vi "Measurement setup.vi"() -> ()   [LabVIEW 2016]
uses:
  Modulation_Signals.ctl
  Modulation_types.ctl
  <vilib>/Utility/config.llb/Write Key (String).vi
  <vilib>/Utility/config.llb/Write Key (Double).vi
  <vilib>/Utility/config.llb/Write Key (Path).vi
  <vilib>/Utility/config.llb/Write Key (Boolean).vi
  <vilib>/Utility/config.llb/Write Key (I32).vi
  <vilib>/Utility/file.llb/Write Delimited Spreadsheet (string).vi
  <vilib>/Utility/file.llb/Write Delimited Spreadsheet (DBL).vi
  <vilib>/Utility/config.llb/NI_LVConfig.lvlib
panel:
  in  "Input channels":cluster{string, "physical channels":tag}[](array[cluster])
  in  "Output channels":cluster{string, "physical channels":tag}[](array[cluster])=[{"ao0", "physical channels"="Dev1/ao0"}, {"ao1", "physical channels"="Dev1/ao1"}]
  in  "Signal param 2":dbl format="%#_6p"
  in  "Mearurement range":dbl=5.0 format="%0.2f"
  in  "High cutoff":dbl=20000.0 format="%#_13p"
  in  "Low cutoff":dbl=20.0 format="%#_13p"
  in  "Filter":bool=TRUE
  out "Export path":path
  in  "Export data":bool
  out "Sampling number":i32
  out "Running":bool
  in  "Resampled iterations":dbl=1.0
  in  "File path":path
  in  "Start":bool
  in  "Modulation type":T1=enum."Simple"
  in  "Modulation signal":T2=enum."Sine"
  out "Output":waveform(dbl)[](graph)
  in  "Modulation depth":dbl=0.8 min=0.0 max=1.000001 step=0.1 format="%0.2f"
  in  "Samples":dbl=200.0 format="%#_12g"
  in  "Signal frequency":dbl=1000.0 format="%#_6p"
  in  "Output Fs":dbl=192000.0 format="%#_6p"
  out "Samples per cycle":dbl=10.0
  in  "Carrier frequency":dbl=40000.0 min=0.0 step=1000.0 format="%#_6p"
  out "data":waveform(dbl)[](graph) caption="Input"
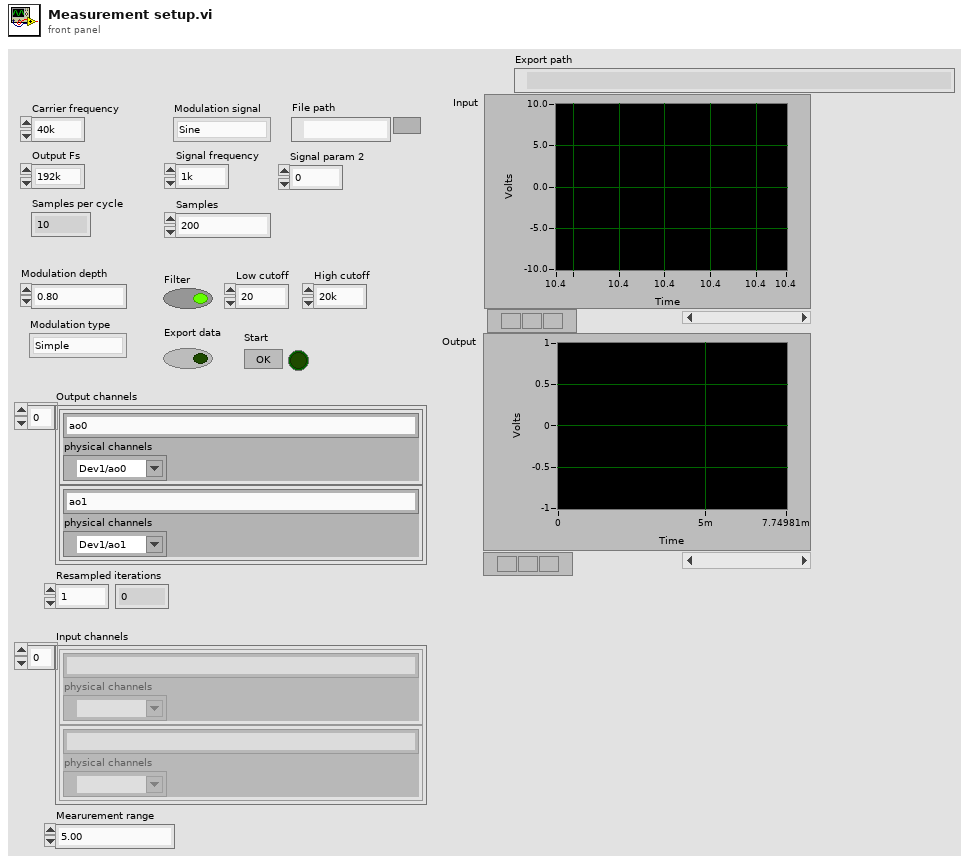
[diagram p1: front panel]
types:
  T1 = typedef "Modulation_types.ctl" = enum16{"None", "Add", "Simple", "Offset", "Square root", "Exponential"}
  T2 = typedef "Modulation_Signals.ctl" = enum16{"None", "Sine", "Chirp", "White Noise", "File"}
  T3 = typedef "NI_LVConfig.lvlib/Config Data RefNum.ctl" = refnum<k1>
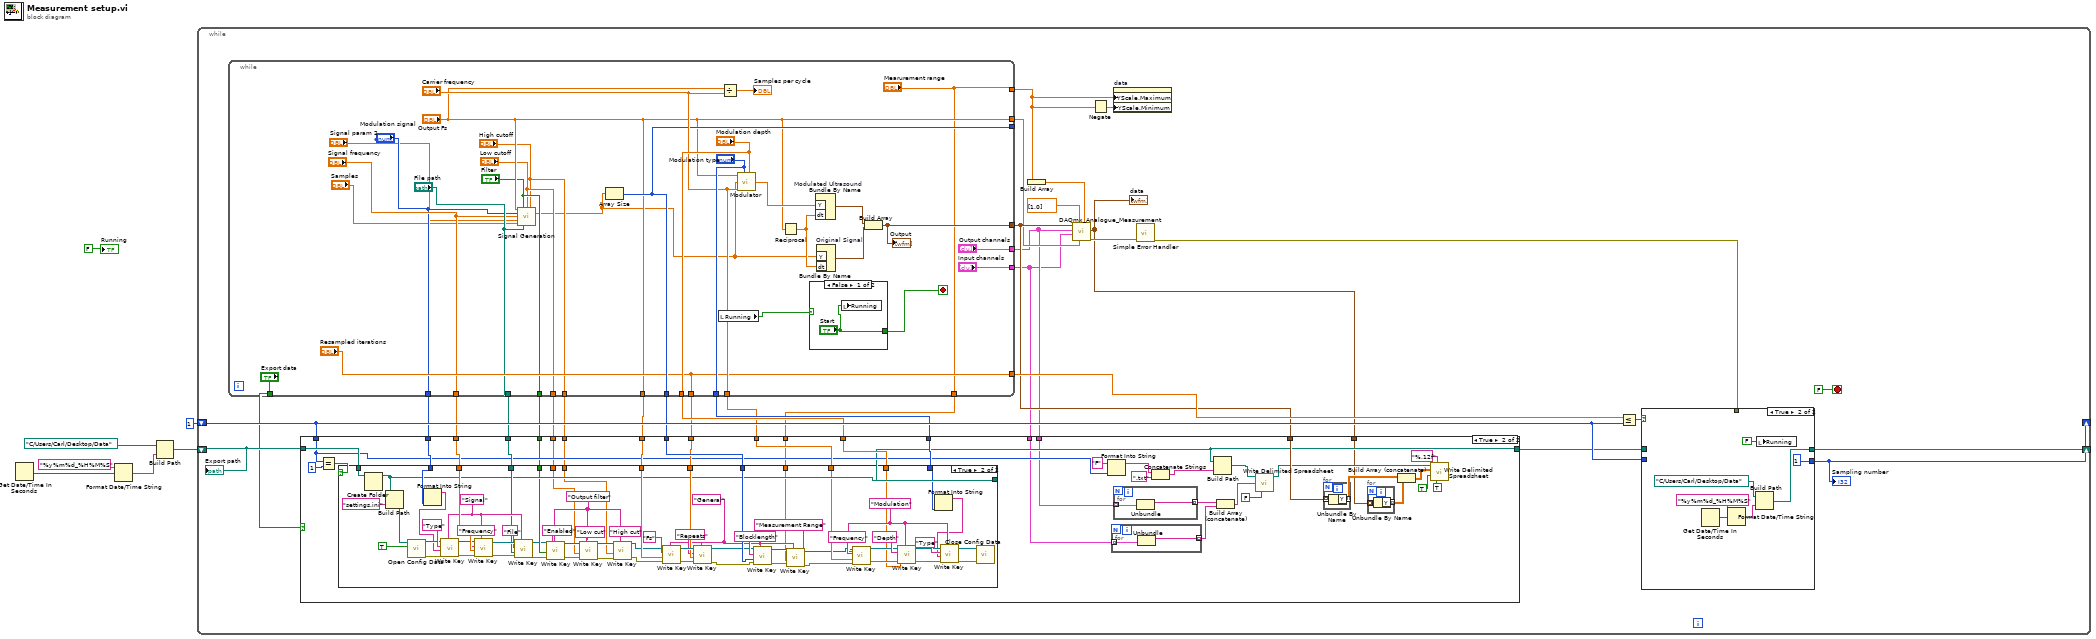
[diagram p0: block diagram]
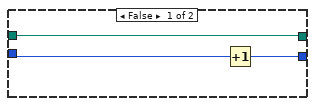
[diagram p4: hidden frame]
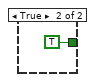
[diagram p5: hidden frame]
diagram:
  n1 = Get Date/Time In Seconds() -> (seconds since 1Jan1904=w6:timestamp)
  n2 = Format Date/Time String(time format string (%c)="%y%m%d_%H%M%S", seconds (now)=w6) -> (date/time string=w5:string)  [unwired: 1 in]
  n3 = Build Path(base path=path "C:/Users/Carl/Desktop/Data", name or relative path=w5) -> (appended path=w2:path)
  n4 = while {
    shift-right: [w39] -> _
    shift-left: 1 ("Sampling number") -> [w38]
    shift-right: [w36] -> _
    shift-left: w2 -> [w35]
    stop <- FALSE stop-if-true
    n5 = while {
      tunnel: [w179] -> _
      tunnel: ["Output Fs"] -> w15
      tunnel: [w187] -> w18
      tunnel: ["Resampled iterations"] -> w19
      tunnel: ["Modulation depth"] -> w34
      tunnel: ["Modulation type"] -> w33
      tunnel: ["Modulation signal"] -> w32
      tunnel: ["Signal frequency"] -> w31
      tunnel: ["File path"] -> w30
      tunnel: ["Carrier frequency"] -> w29
      tunnel: ["Output Fs"] -> w28
      tunnel: [w179] -> w27
      tunnel: ["Resampled iterations"] -> w26
      tunnel: ["Export data"] -> w25
      tunnel: ["Mearurement range"] -> w13
      tunnel: ["Mearurement range"] -> w24
      tunnel: ["Filter"] -> w23
      tunnel: ["Low cutoff"] -> w22
      tunnel: ["High cutoff"] -> w21
      tunnel: ["Output channels"] -> w9
      tunnel: ["Input channels"] -> w8
      stop <- w184 stop-if-true
      n6 = call "Signal Generation.vi"("Output Fs"="Output Fs", "Filter"="Filter", "Low cutoff"="Low cutoff", "High cutoff"="High cutoff", "Signal Type"="Modulation signal", "Frequency 1"="Signal frequency", "Frequency 2"="Signal param 2", "Samples"="Samples", "File path"="File path") -> ("Output Signal"=w164:dbl[])  [unwired: 6 in]
      n7 = Array Size(array=w164) -> (size(s)=w179:i32)
      n8 = local read "Running"() -> (w183:bool)
      n9 = Divide(x="Output Fs", y="Carrier frequency") -> (x/y=→"Samples per cycle":dbl)
      n10 = call "Modulator.vi"("Sampling frequency"="Output Fs", "Modulation Type"="Modulation type", "Input Signal"=w164, "Carrier Frequency"="Carrier frequency", "Modulation depth"="Modulation depth") -> ("Output signal"=w188:dbl[])  [unwired: 4 in]
      n11 = Reciprocal(x="Output Fs") -> (1/x=w189:dbl)
      n12 = case shown="False" w183 {
        tunnel: ["Start" TRUE ("Start")] -> w184
        frame False {
          n13 = local write "Running"("Start") -> ()
        }
        frame True {
        }
      }
      n14 = Bundle By Name "Modulated Ultrasound"("Y"=w188, "dt"=w189) -> (w185:waveform(dbl))  [unwired: 1 in]
      n15 = Bundle By Name "Original Signal"("Y"=w164, "dt"=w189) -> (w190:waveform(dbl))  [unwired: 1 in]
      n16 = Build Array(w185, w190) -> (w187:waveform(dbl)[])
      "Output" <- w187
    }
    n17 = Build Array(w13) -> (w16:dbl[])
    n18 = call "DAQmx_Analogue_Measurement.vi"("Input ranges"=w16, "Sampling rate"=w15, "Output ranges"=dbl[] [1.0], "Input channels"=w8, "Output channels"=w9, "Outputs"=w18) -> ("error out"=w12:errorcluster, "Measured data"=w11:waveform(dbl)[])  [unwired: 4 in]
    "data" <- w11
    n19 = case shown="True" w25 {
      tunnel: w38 -> [_ w67]
      tunnel: w35 -> [w41 w68]
      tunnel: [w41 w58] -> w37
      tunnel: w34 -> [_ w77]
      tunnel: w33 -> [_ w76]
      tunnel: w32 -> [_ w75]
      tunnel: w31 -> [_ w74]
      tunnel: w30 -> [_ w73]
      tunnel: w29 -> [_ w72]
      tunnel: w28 -> [_ w71]
      tunnel: w27 -> [_ w70]
      tunnel: w26 -> [_ w69]
      tunnel: w18 -> [_ w63]
      tunnel: w24 -> [_ w56]
      tunnel: w23 -> [_ w55]
      tunnel: w22 -> [_ w54]
      tunnel: w21 -> [_ w53]
      tunnel: w11 -> [_ w46]
      tunnel: w9 -> [_ w45]
      tunnel: w8 -> [_ w44]
      frame False {
      }
      frame True {
        n20 = Equal?(x=w67, y=1) -> (x = y?=w78:bool)
        n21 = case shown="True" w78 {
          tunnel: w68 -> [w88 w114]
          tunnel: w77 -> [_ w99]
          tunnel: w76 -> [_ w118]
          tunnel: w75 -> [_ w120]
          tunnel: w74 -> [_ w141]
          tunnel: w73 -> [_ w134]
          tunnel: w72 -> [_ w98]
          tunnel: w71 -> [_ w131]
          tunnel: w70 -> [_ w130]
          tunnel: w69 -> [_ w126]
          tunnel: [w88 w113] -> w58
          tunnel: w56 -> [_ w108]
          tunnel: w55 -> [_ w95]
          tunnel: w54 -> [_ w94]
          tunnel: w53 -> [_ w93]
          frame False {
          }
          frame True {
            w103 = "Output filter" ("section")
            w110 = "General"
            w137 = "Signal" ("section")
            w132 = "Modulation" ("section")
            n22 = Create Folder(path (use dialog)=w114) -> (created path=w113:path)  [unwired: 2 in, 2 out]
            n23 = Build Path(base path=w113, name or relative path="settings.ini") -> (appended path=w116:path)
            n24 = call <vilib>:"Open Config Data.vi"("create file if necessary (T)"=TRUE, "configuration file path"=w116) -> ("error out"=w143:errorcluster, "refnum"=w142:T3)  [unwired: 7 in, 1 out]
            n25 = Format Into String(w120) -> (resulting string=w119:string)  [unwired: 3 in, 1 out]
            n26 = call-poly <vilib>:"Write Key.vi"("section"=w137, "error in (no error)"=w143, "value"=w119, "key"="Type", "refnum"=w142) -> ("error out"=w139:errorcluster, "refnum out"=w138:T3)  [unwired: 4 in, 1 out]
            n27 = call-poly <vilib>:"Write Key.vi"("section"=w137, "error in (no error)"=w139, "value"=w141, "key"="Frequency", "refnum"=w138) -> ("error out"=w135:errorcluster, "refnum out"=w136:T3)  [unwired: 4 in, 1 out]
            n28 = call-poly <vilib>:"Write Key.vi"("section"=w137, "error in (no error)"=w135, "value"=w134, "key"="File", "refnum"=w136) -> ("error out"=w90:errorcluster, "refnum out"=w89:T3)  [unwired: 4 in, 1 out]
            n29 = call-poly <vilib>:"Write Key.vi"("section"=w103, "error in (no error)"=w90, "value"=w95, "key"="Enabled", "refnum"=w89) -> ("error out"=w107:errorcluster, "refnum out"=w106:T3)  [unwired: 4 in, 1 out]
            n30 = call-poly <vilib>:"Write Key.vi"("section"=w103, "error in (no error)"=w107, "value"=w94, "key"="Low cut", "refnum"=w106) -> ("error out"=w104:errorcluster, "refnum out"=w105:T3)  [unwired: 4 in, 1 out]
            n31 = call-poly <vilib>:"Write Key.vi"("section"=w103, "error in (no error)"=w104, "value"=w93, "key"="High cut", "refnum"=w105) -> ("error out"=w92:errorcluster, "refnum out"=w91:T3)  [unwired: 4 in, 1 out]
            n32 = call-poly <vilib>:"Write Key.vi"("section"=w110, "error in (no error)"=w92, "value"=w131, "key"="Fs", "refnum"=w91) -> ("error out"=w128:errorcluster, "refnum out"=w127:T3)  [unwired: 4 in, 1 out]
            n33 = call-poly <vilib>:"Write Key.vi"("section"=w110, "error in (no error)"=w128, "value"=w126, "key"="Repeats", "refnum"=w127) -> ("error out"=w124:errorcluster, "refnum out"=w123:T3)  [unwired: 4 in, 1 out]
            n34 = call-poly <vilib>:"Write Key.vi"("section"=w110, "error in (no error)"=w124, "value"=w130, "key"="Blocklength", "refnum"=w123) -> ("error out"=w112:errorcluster, "refnum out"=w111:T3)  [unwired: 4 in, 1 out]
            n35 = call-poly <vilib>:"Write Key.vi"("section"=w110, "error in (no error)"=w112, "value"=w108, "key"="Measurement Range", "refnum"=w111) -> ("error out"=w96:errorcluster, "refnum out"=w97:T3)  [unwired: 4 in, 1 out]
            n36 = call-poly <vilib>:"Write Key.vi"("section"=w132, "error in (no error)"=w96, "value"=w98, "key"="Frequency", "refnum"=w97) -> ("error out"=w148:errorcluster, "refnum out"=w149:T3)  [unwired: 4 in, 1 out]
            n37 = call-poly <vilib>:"Write Key.vi"("section"=w132, "error in (no error)"=w148, "value"=w99, "key"="Depth", "refnum"=w149) -> ("error out"=w146:errorcluster, "refnum out"=w145:T3)  [unwired: 4 in, 1 out]
            n38 = Format Into String(w118) -> (resulting string=w117:string)  [unwired: 3 in, 1 out]
            n39 = call-poly <vilib>:"Write Key.vi"("section"=w132, "error in (no error)"=w146, "value"=w117, "key"="Type", "refnum"=w145) -> ("error out"=w121:errorcluster, "refnum out"=w122:T3)  [unwired: 4 in, 1 out]
            n40 = call <vilib>:"Close Config Data.vi"("error in (no error)"=w121, "refnum"=w122) -> ()  [unwired: 8 in, 2 out]
          }
        }
        n41 = Format Into String(initial string="F", w67) -> (resulting string=w66:string)  [unwired: 2 in, 1 out]
        n42 = for {
          tunnel: w44 -> [w83] mode=indexing
          tunnel: [w82] -> w42 mode=indexing
          n43 = Unbundle(w83) -> (w82:string)  [unwired: 1 out]
        }
        n44 = for {
          tunnel: w45 -> [w81] mode=indexing
          tunnel: [w80] -> w43 mode=indexing
          n45 = Unbundle(w81) -> (w80:string)  [unwired: 1 out]
        }
        n46 = Concatenate Strings(w66, ".txt" ("string")) -> (w64:string)
        n47 = Build Path(base path=w58, name or relative path=w64) -> (appended path=w52:path)
        n48 = Build Array (concatenate)(w43, w42) -> (w50:string[])
        n49 = call-poly <vilib>:"Write Delimited Spreadsheet.vi"("file path (dialog if empty)"=w52, "1D data"=w50, "transpose? (no:F)"=FALSE) -> ("new file path (Not A Path if cancelled)"=w51:path)  [unwired: 11 in, 1 out]
        n50 = for {
          tunnel: w63 -> [w87] mode=indexing
          tunnel: [w86] -> w60 mode=indexing
          n51 = Unbundle By Name(w87) -> ("Y"=w86:dbl[])
        }
        n52 = for {
          tunnel: [w85] -> w61 mode=indexing
          tunnel: w46 -> [w84] mode=indexing
          n53 = Unbundle By Name(w84) -> ("Y"=w85:dbl[])
        }
        n54 = Build Array (concatenate)(w60, w61) -> (w59:dbl[][])
        n55 = call-poly <vilib>:"Write Delimited Spreadsheet.vi"("file path (dialog if empty)"=w51, "format (%.3f)"="%.12f", "2D data"=w59, "append to file? (new file:F)"=TRUE, "transpose? (no:F)"=TRUE) -> ()  [unwired: 9 in, 2 out]
      }
    }
    n56 = Negate(x=w13) -> (-x=w14:dbl)
    n57 = property on="data" class="WFGraph (strict)"("YScale.Maximum"=w13, "YScale.Minimum"=w14) -> ()  [unwired: 2 in, 2 out]
    n58 = call <vilib>:"Simple Error Handler.vi"("error in (no error)"=w12) -> ("error out"=w20:errorcluster)  [unwired: 4 in, 4 out]
    n59 = Less Or Equal?(x=w19, y=w38) -> (x <= y?=w10:bool)
    n60 = case shown="True" w10 {
      tunnel: w38 -> [w156 _]
      tunnel: [w155 1 ("Sampling number")] -> w39
      tunnel: w20 -> [_ _]
      tunnel: [w154 w157] -> w36
      tunnel: w37 -> [w154 _]
      frame False {
        n61 = Increment(x=w156) -> (x+1=w155:i32)
      }
      frame True {
        n62 = Get Date/Time In Seconds() -> (seconds since 1Jan1904=w161:timestamp)
        n63 = Format Date/Time String(time format string (%c)="%y%m%d_%H%M%S", seconds (now)=w161) -> (date/time string=w160:string)  [unwired: 1 in]
        n64 = Build Path(base path=path "C:/Users/Carl/Desktop/Data", name or relative path=w160) -> (appended path=w157:path)
        n65 = local write "Running"(FALSE ("Running")) -> ()
      }
    }
    "Sampling number" <- w39
    "Export path" <- w35
  }
  "Running" <- FALSE
